vi "testCOPY.vi"(7 "error in":errorcluster) -> (20 "Matches (Geometric Matching 1)":T2[](array[typedef]) {"Correlation Score" format="%.2f"; "Target Template Curve Score" format="%.2f"; "Template Target Curve Score" format="%.2f"; "Bounding Box"."y" format="%.2f"; "Bounding Box"."x" format="%.2f"; "Position"."y" format="%.2f"; "Position"."x" format="%.2f"; "Score" format="%.2f"; "Scale" format="%.2f"; "Angle" format="%.2f"; "Occlusion %" format="%.2f"}, 21 "Calibrated Matches (Geometric Matching 1)":T2[](array[typedef]) {"Correlation Score" format="%.2f"; "Target Template Curve Score" format="%.2f"; "Template Target Curve Score" format="%.2f"; "Bounding Box"."y" format="%.2f"; "Bounding Box"."x" format="%.2f"; "Position"."y" format="%.2f"; "Position"."x" format="%.2f"; "Score" format="%.2f"; "Scale" format="%.2f"; "Angle" format="%.2f"; "Occlusion %" format="%.2f"}, 22 "Number of Matches (Geometric Matching 1)":i32, 27 "error out":errorcluster)   [LabVIEW 2016]
uses:
  <vilib>/vision/Pattern Matching.llb/IMAQ GM Match Report.ctl
  <vilib>/vision/Pattern Matching.llb/IMAQ Curve Parameters.ctl
  <vilib>/vision/Pattern Matching.llb/IMAQ Match Range Setting.ctl
  <vilib>/vision/NI_Vision_Development_Module.lvlib
panel:
  out "Image Out":T1(plugin-control)
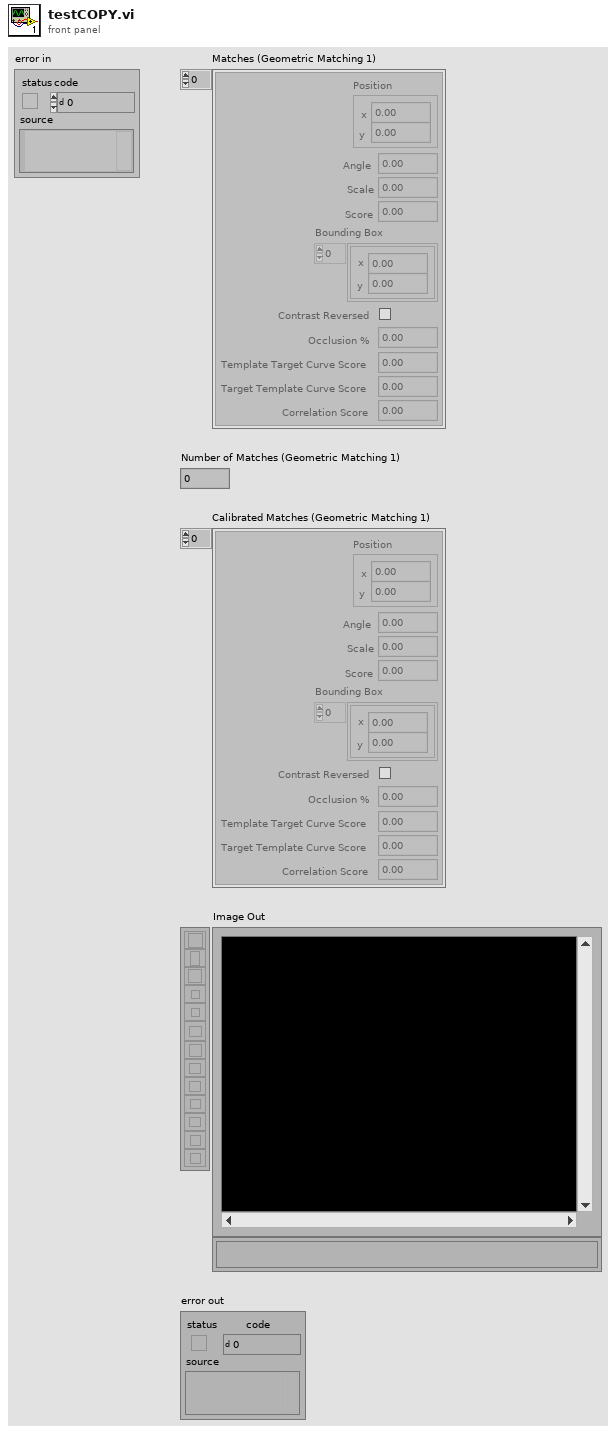
[diagram p1: front panel]
types:
  T1 = typedef "IMAQ Image.ctl" = refnum<image>
  T2 = typedef "IMAQ GM Match Report.ctl" = cluster{"Position":cluster{"x":sgl, "y":sgl}, "Angle":sgl, "Scale":sgl, "Score":sgl, "Bounding Box":cluster{"x":sgl, "y":sgl}[], "Contrast Reversed":bool, "Occlusion %":sgl, "Template Target Curve Score":sgl, "Target Template Curve Score":sgl, "Correlation Score":sgl}
  T3 = typedef "IMAQ Curve Parameters.ctl" = cluster{"Extraction Mode":u32, "Edge Threshold":i32, "Edge Filter Size":u32, "Min Length":i32, "Row Search Step Size":i32, "Col Search Step Size":i32, "Max Endpoint Gap":i32, "Closed":bool, "Subpixel":bool}
  T4 = typedef "IMAQ Match Range Setting.ctl" = cluster{"Match Constraints":u32, "Min":dbl, "Max":dbl}
  T5 = cluster{"Curve Parameters":T3, "Match Mode":cluster{"Rotation":bool, "Scale":bool, "Occlusion":bool, "Reserved":bool, "Reserved":bool, "Reserved":bool}, "Range Settings":T4[], "Number of Matches":i32, "Minimum Match Score":sgl, "SubPixel Accuracy":bool, "Adv. Geometric Match Options 2":cluster{"Setup Data Item":u16, "Item Value":dbl}[]}
  T6 = cluster{"Global Rectangle":i32[], "Contours":cluster{"ID":enum32{"External", "Internal"}, "Type":u32, "Coordinates":i32[]}[]}
  T7 = cluster{"Brightness":sgl, "Contrast":sgl, "Gamma":sgl}
  T8 = typedef "Image Type" = u32
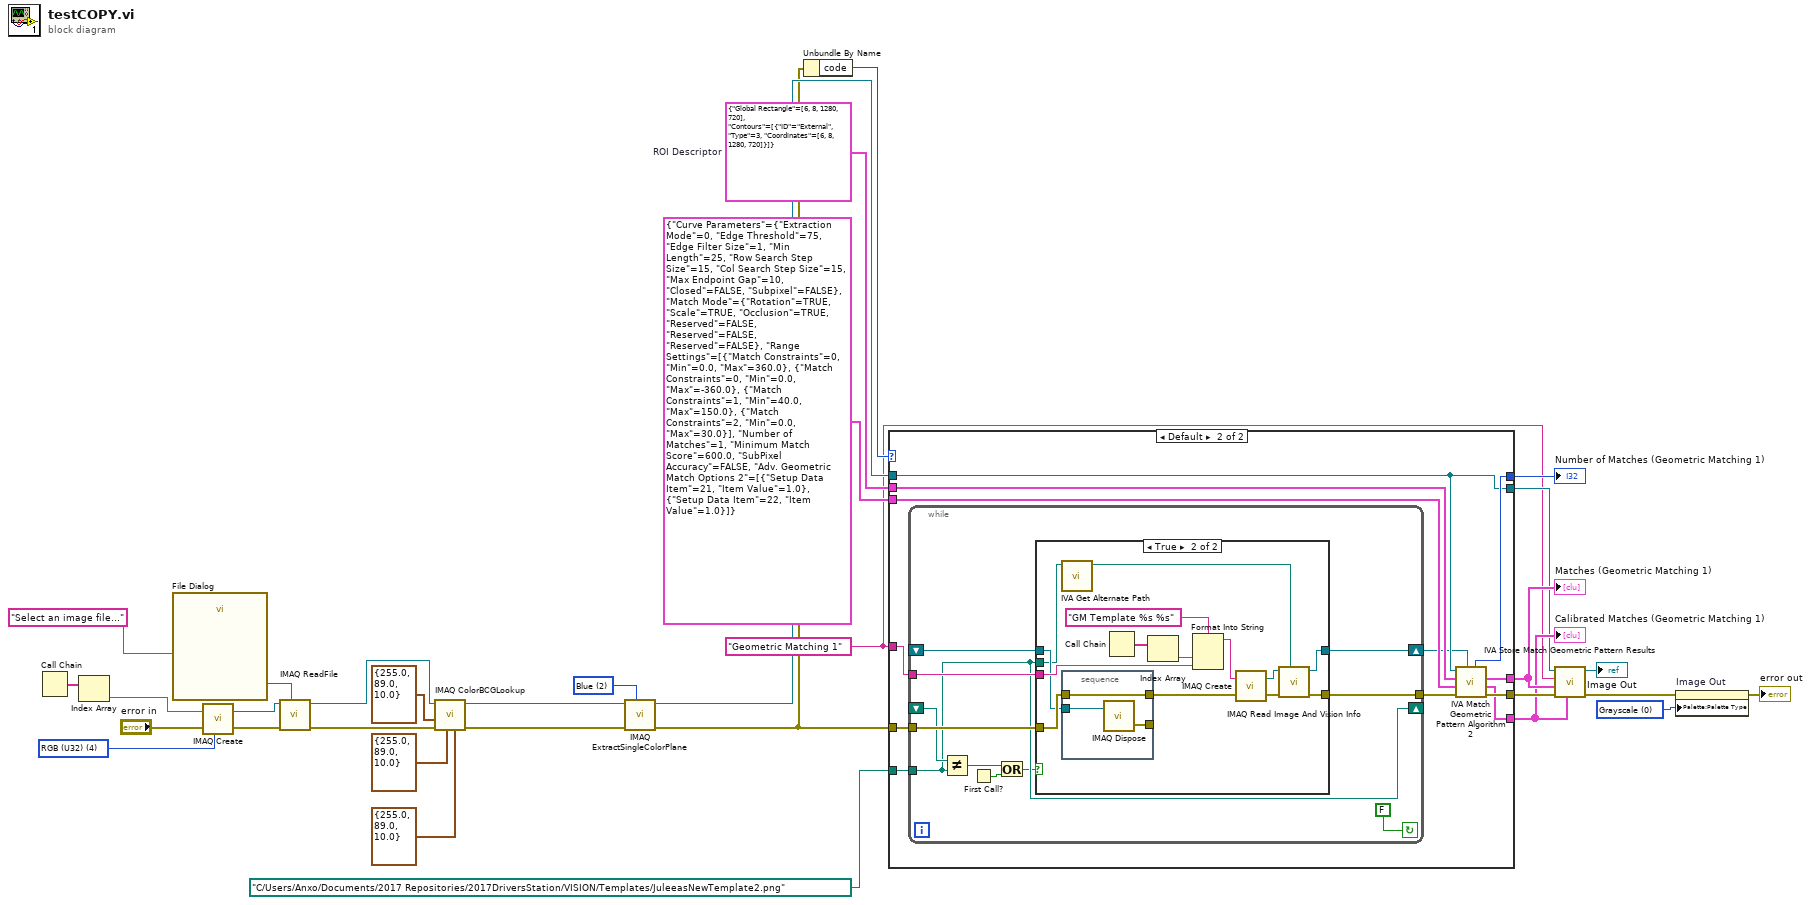
[diagram p0: block diagram]
diagram:
  w1 = u32 0 items=["Grayscale", "Binary", "Gradient", "Rainbow", "Temperature", "User Defined", "Binary 16 Bit", "Gradient 16 Bit", "Rainbow 16 Bit", "Temperature 16 Bit", "User Defined 16 Bit"] ("Palette Type")
  w5 = "Geometric Matching 1" ("Step Name")
  w15 = T6 {"Global Rectangle"=[6, 8, 1280, 720], "Contours"=[{"ID"=enum."External", "Type"=3, "Coordinates"=[6, 8, 1280, 720]}]}  # ROI Descriptor
  w19 = 2 items=["Red", "Green", "Blue", "Hue", "Saturation", "Luminance", "Value", "Intensity"] ("Color Plane")
  w25 = T8 4 items=["Grayscale (U8)", "Grayscale (I16)", "Grayscale (SGL)", "Complex (CSG)", "RGB (U32)", "HSL (U32)", "RGB (U64)", "Grayscale (U16)"] ("Image Type")
  n1 = Call Chain() -> (call chain=w29:string[])
  n2 = Index Array(array=w29) -> (element=w28:string)  [unwired: 1 in]
  n3 = call "File Dialog"("prompt"="Select an image file...") -> ("selected path"=w26:path)  [unwired: 6 in, 8 out]
  n4 = call "IMAQ Create"("Image Name"=w28, "Image Type"=w25, "error in (no error)"="error in") -> ("New Image"=w32:T1, "error out"=w31:errorcluster)  [unwired: 1 in, 1 out]
  n5 = call "IMAQ ReadFile"("File Path"=w26, "error in (no error)"=w31, "Image"=w32) -> ("error out"=w23:errorcluster, "Image Out"=w24:T1)  [unwired: 2 in, 5 out]
  n6 = call "IMAQ ColorBCGLookup"("Blue BCG Values"=T7 {"Brightness"=255.0, "Contrast"=89.0, "Gamma"=10.0}, "Green BCG Values"=T7 {"Brightness"=255.0, "Contrast"=89.0, "Gamma"=10.0}, "error in (no error)"=w23, "Red BCG Values"=T7 {"Brightness"=255.0, "Contrast"=89.0, "Gamma"=10.0}, "Image Src"=w24) -> ("error out"=w17:errorcluster, "Image Dst Out"=w18:T1)  [unwired: 2 in, 3 out]
  n7 = call "IMAQ ExtractSingleColorPlane"("Color Plane"=w19, "error in (no error)"=w17, "Image Src"=w18) -> ("error out"=w9:errorcluster, "Image Dst Out"=w14:T1)  [unwired: 1 in, 6 out]
  n8 = Unbundle By Name(w9) -> ("code"=w8:i32)
  n9 = case shown="Default" w8 {
    tunnel: path "C:/Users/Anxo/Documents/2017 Repositories/2017DriversStation/VISION/Templates/JuleeasNewTemplate2.png" ("Template File Path") -> [_ w38]
    tunnel: w9 -> [_ w37]
    tunnel: T5 {"Curve Parameters"={"Extraction Mode"=0, "Edge Threshold"=75, "Edge Filter Size"=1, "Min Length"=25, "Row Search Step Size"=15, "Col Search Step Size"=15, "Max Endpoint Gap"=10, "Closed"=FALSE, "Subpixel"=FALSE}, "Match Mode"={"Rotation"=TRUE, "Scale"=TRUE, "Occlusion"=TRUE, "Reserved"=FALSE, "Reserved"=FALSE, "Reserved"=FALSE}, "Range Settings"=[{"Match Constraints"=0, "Min"=0.0, "Max"=360.0}, {"Match Constraints"=0, "Min"=0.0, "Max"=-360.0}, {"Match Constraints"=1, "Min"=40.0, "Max"=150.0}, {"Match Constraints"=2, "Min"=0.0, "Max"=30.0}], "Number of Matches"=1, "Minimum Match Score"=600.0, "SubPixel Accuracy"=FALSE, "Adv. Geometric Match Options 2"=[{"Setup Data Item"=21, "Item Value"=1.0}, {"Setup Data Item"=22, "Item Value"=1.0}]} ("Settings") -> [_ w45]
    tunnel: w15 -> [_ w44]
    tunnel: w14 -> [w33 w39]
    tunnel: [_ w43] -> w13
    tunnel: [_ w42] -> w12
    tunnel: [_ w41] -> w11
    tunnel: [_ w40] -> w10
    tunnel: [w33 w39] -> w7
    tunnel: w5 -> [_ w34]
    frame -1074396199, -1074396198 {
      # "Discard Coordinate System Error"
    }
    frame Default {
      n10 = while {
        shift-right: [w56] -> w35
        shift-left: _ -> [w55]
        tunnel: [w53] -> w36
        tunnel: w37 -> [w52]
        tunnel: w38 -> [w49]
        tunnel: w34 -> [w51]
        shift-right: [w49] -> _
        shift-left: _ -> [w50]
        stop <- FALSE continue-if-true
        n11 = Not Equal?(x=w50, y=w49) -> (x != y?=w47:bool)
        n12 = First Call?() -> (First Call?: T/F=w48:bool)
        n13 = Or(x=w47, y=w48) -> (x .or. y?=w46:bool)
        n14 = case shown="True" w46 {
          tunnel: [w58 w70] -> w56
          tunnel: w55 -> [w58 w62]
          tunnel: [w57 w67] -> w53
          tunnel: w52 -> [w57 w63]
          tunnel: w51 -> [_ w64]
          tunnel: w49 -> [_ w60]
          frame False {
          }
          frame True {
            n15 = call <vilib>:"IVA Get Alternate Path.vi"("Path In"=w60) -> ("Path Out"=w59:path)  [unwired: 10 out]
            n16 = stacked-sequence {
              tunnel: w63 -> [w75]
              tunnel: w62 -> [w74]
              tunnel: [w75] -> w61
              tunnel: [w73] -> _
              frame #0 {
                n17 = call "IMAQ Dispose"("Image"=w74) -> ("error out"=w73:errorcluster)  [unwired: 2 in, 3 out]
              }
            }
            n18 = Call Chain() -> (call chain=w66:string[])
            n19 = Index Array(array=w66) -> (element=w65:string)  [unwired: 1 in]
            n20 = Format Into String(format string="GM Template %s %s" ("Image Name"), w65, w64) -> (resulting string=w72:string)  [unwired: 2 in, 1 out]
            n21 = call "IMAQ Create"("Image Name"=w72, "error in (no error)"=w61) -> ("New Image"=w69:T1, "error out"=w68:errorcluster)  [unwired: 2 in, 1 out]
            n22 = call "IMAQ Read Image And Vision Info"("File Path"=w59, "error in (no error)"=w68, "Image"=w69) -> ("error out"=w67:errorcluster, "Image Out"=w70:T1)  [unwired: 1 in, 6 out]
          }
        }
      }
      n23 = call <vilib>:"IVA Match Geometric Pattern Algorithm 2.vi"("Template"=w35, "error in (no error)"=w36, "Settings"=w45, "ROI Descriptor"=w44, "Image"=w39) -> ("error out"=w43:errorcluster, "Calibrated Matches"=w41:T2[], "Matches"=w42:T2[], "Number of Matches"=w40:i32)  [unwired: 1 in, 2 out]
    }
  }
  "Matches (Geometric Matching 1)" <- w12
  "Number of Matches (Geometric Matching 1)" <- w10
  "Calibrated Matches (Geometric Matching 1)" <- w11
  n24 = call <vilib>:"IVA Store Match Geometric Pattern Results.vi"("Calibrated Matches"=w11, "error in (no error)"=w13, "Matches"=w12, "Step Name"=w5, "Image in"=w7) -> ("error out"=w4:errorcluster, "Image dup"=→"Image Out":T1)  [unwired: 5 out]
  n25 = property on="Image Out" class="ImageControl"(error in=w4, "Palette:Palette Type"=w1) -> (error out=→"error out":errorcluster)  [unwired: 1 in, 1 out]
